vi "Initialize_Array_2D.vi"(9 "Value":i8, 10 "Dimensions":T1 {"Columns" min=0; "Rows" min=0}) -> (2 "Initialized Array 2D":i8[][](array[numeric]))   [LabVIEW 2018]
uses:
  Controls/Rows_Columns.ctl
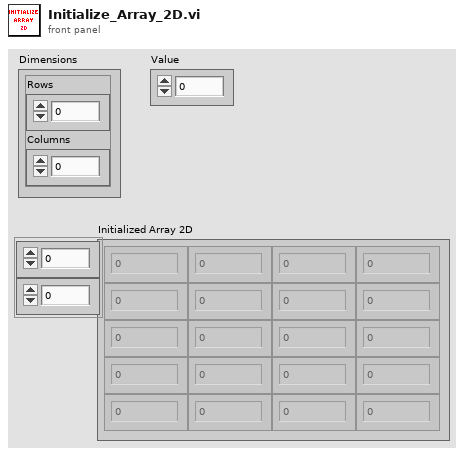
[diagram p1: front panel]
types:
  T1 = typedef "Rows_Columns.ctl" = cluster{"Rows":i32, "Columns":i32}
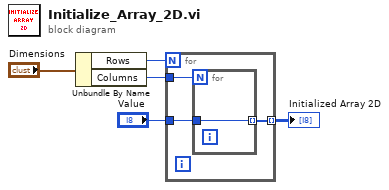
[diagram p0: block diagram]
diagram:
  n1 = Unbundle By Name("Dimensions") -> ("Rows"=w2:i32, "Columns"=w1:i32)
  n2 = for {
    N: w2 -> [_]
    tunnel: "Value" -> [w8]
    tunnel: [w7] -> w5 mode=indexing
    tunnel: w1 -> [w6]
    n3 = for {
      N: w6 -> [_]
      tunnel: [w9] -> w7 mode=indexing
      tunnel: w8 -> [w9]
    }
  }
  "Initialized Array 2D" <- w5
